vi "Calculate Distance of differences.vi"(10 "Column Differences":i32[](array[numeric]), 11 "Row Differences":i32[](array[numeric])) -> (3 "Array 3":dbl[](array[numeric]))   [LabVIEW 2016, in "AntFarm_MB.lvclass"]
uses:
  AntFarm_MB.lvclass
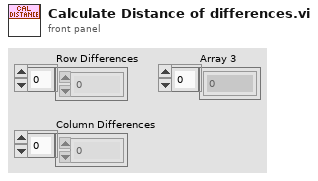
[diagram p1: front panel]
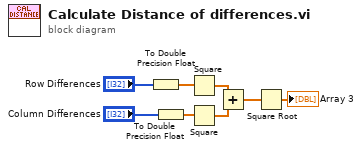
[diagram p0: block diagram]
diagram:
  n1 = To Double Precision Float(number="Row Differences") -> (double precision float=w1:dbl[])
  n2 = To Double Precision Float(number="Column Differences") -> (double precision float=w2:dbl[])
  n3 = Square(x=w1) -> (x^2=w3:dbl[])
  n4 = Square(x=w2) -> (x^2=w4:dbl[])
  n5 = Add(x=w3, y=w4) -> (x+y=w5:dbl[])
  n6 = Square Root(x=w5) -> (sqrt(x)=→"Array 3":dbl[])
